vi "UnregisterAppender.vi"(8 "error in (no error)":errorcluster, 10 "id":string, 11 "Logger in":refnum<class "Logger.lvclass">) -> (0 "error out":errorcluster, 3 "Logger out":refnum<class "Logger.lvclass">)   [LabVIEW 2026, in "Lumberjack.lvlib" / "Logger.lvclass"]
uses:
  Logger.lvclass
  Logger.lvclass/Logger.ctl
  TypeDefs/SnapshotWaitMode.ctl
  <vilib>/ActorFramework/Message Enqueuer/Message Enqueuer.lvclass
  Core/Messages/UnregisterAppenderMsg.lvclass/UnregisterAppenderMsg.lvclass
  Lumberjack.lvlib
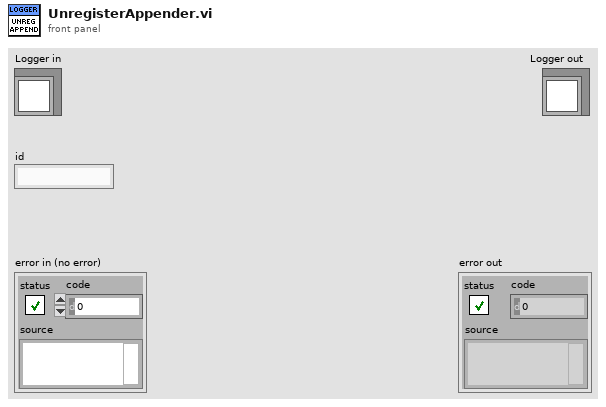
[diagram p1: front panel]
types:
  T1 = typedef "Lumberjack.lvlib/SnapshotWaitMode.ctl" = enum16{"AnySnapshot", "IDPresent", "IDAbsent"}
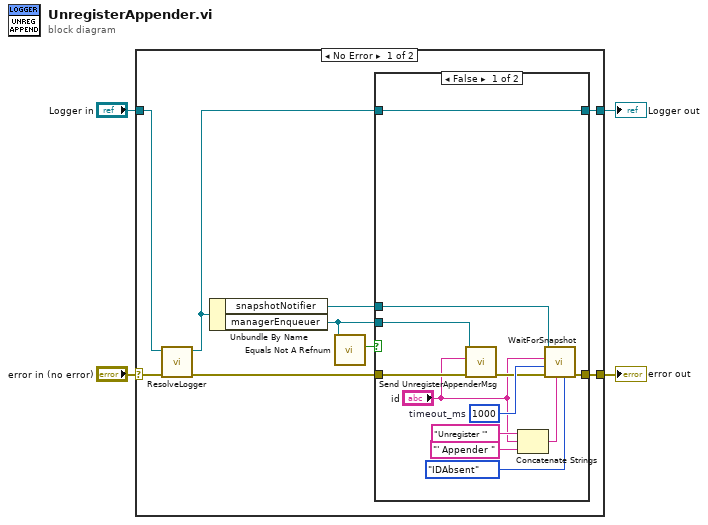
[diagram p0: block diagram]
diagram:
  n1 = case shown="No Error" "error in (no error)" {
    selector: "error in (no error)" -> [w13 w29]
    tunnel: [w11 w29] -> w3
    tunnel: [w9 w28] -> w1
    tunnel: "Logger in" -> [w10 w28]
    frame No Error {
      n2 = call "ResolveLogger.vi"("error in (no error)"=w13, "Logger in"=w10) -> ("error out"=w12:errorcluster, "Logger out"=w8:refnum<class "Logger.lvclass">)  [unwired: 8 in]
      n3 = Unbundle By Name(w8) -> ("snapshotNotifier"=w5:refnum<notifier>, "managerEnqueuer"=w6:refnum<class "Message Enqueuer.lvclass">)
      n4 = call <vilib>:"Equals Not A Refnum.vi"("Message Enqueuer"=w6) -> ("Not a refnum?"=w7:bool)  [unwired: 10 in]
      n5 = case shown="False" w7 {
        tunnel: w12 -> [w24 w27]
        tunnel: [w19 w27] -> w11
        tunnel: [w25 w26] -> w9
        tunnel: w8 -> [w25 w26]
        tunnel: w6 -> [w23 _]
        tunnel: w5 -> [w14 _]
        frame False {
          w22 = 1000  # timeout_ms
          n6 = call "Send UnregisterAppenderMsg.vi"("error in (no error)"=w24, "id"="id", "Enqueuer in"=w23) -> ("error out"=w20:errorcluster)  [unwired: 7 in, 1 out]
          n7 = Concatenate Strings("Unregister '" ("Context"), "id", "' Appender " ("Context")) -> (w15:string)
          n8 = call "WaitForSnapshot.vi"("SnapshotWaitMode"=SnapshotWaitMode."IDAbsent", "Context"=w15, "error in (no error)"=w20, "timeout_ms"=w22, "targetID"="id", "notifier"=w14) -> ("error out"=w19:errorcluster)  [unwired: 4 in, 1 out]
        }
        frame True {
        }
      }
    }
    frame Error {
    }
  }
  "error out" <- w3
  "Logger out" <- w1
